vi "InsertBehavior.vi"(7 "exp_type":string, 8 "error in (no error)":errorcluster, 9 "beh_path":path, 10 "beh_start_time":timestamp, 11 "connection reference":T1) -> (0 "error out":errorcluster, 3 "BehaviorPK":T2)   [LabVIEW 2010]
uses:
  <vilib>/addons/database/NI_Database_API.lvlib
  BehPrimary.ctl
  SessionPrimary.ctl
  <vilib>/addons/database/Connection.llb/Conn ObjectReference.ctl
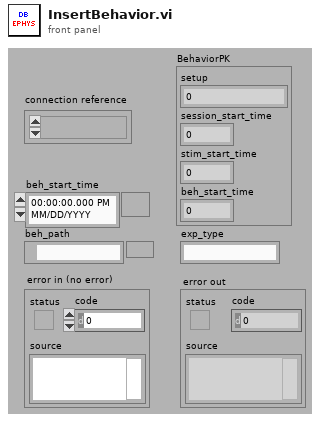
[diagram p1: front panel]
types:
  T1 = typedef "NI_Database_API.lvlib/Conn ObjectReference.ctl" = refnum<k1>
  T2 = typedef "BehPrimary.ctl" = cluster{"setup":u8, "session_start_time":dbl, "stim_start_time":dbl, "beh_start_time":dbl}
  T3 = cluster{"setup":u8, "session_start_time":timestamp, "beh_start_time":timestamp, "beh_path":path, "exp_type":string}
  T4 = typedef "SessionPrimary.ctl" = cluster{"setup":u8, "session_start_time":dbl}
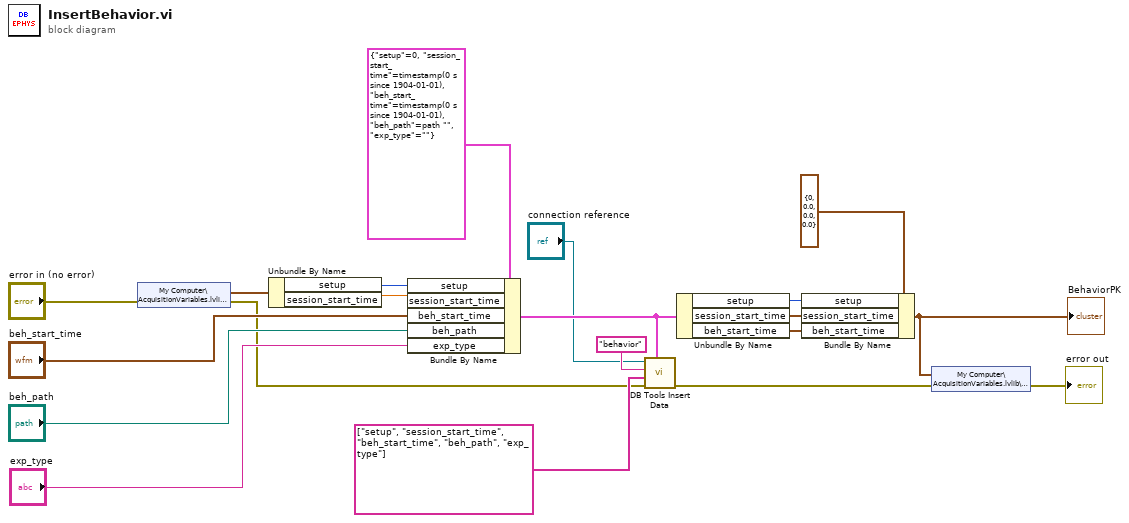
[diagram p0: block diagram]
diagram:
  n1 = shared-variable "My Computer\\AcquisitionVariables.lvlib\\SessionPK"(error in="error in (no error)") -> (w6:T4, error out=w4:errorcluster)
  n2 = Unbundle By Name(w6) -> ("setup"=w17:u8, "session_start_time"=w16:dbl)
  n3 = Bundle By Name(cluster=T3 {"setup"=0, "session_start_time"=timestamp(0 s since 1904-01-01), "beh_start_time"=timestamp(0 s since 1904-01-01), "beh_path"=path "", "exp_type"=""} ("Cluster"), "setup"=w17, "session_start_time"=w16, "beh_start_time"="beh_start_time", "beh_path"="beh_path", "exp_type"="exp_type") -> (w13:T3)
  n4 = call <vilib>:"DB Tools Insert Data.vi"("data"=w13, "error in (no error)"=w4, "columns"=string[] ["setup", "session_start_time", "beh_start_time", "beh_path", "exp_type"], "table"="behavior", "connection reference"="connection reference") -> ("error out"=w2:errorcluster)  [unwired: 5 in, 1 out]
  n5 = Unbundle By Name(w13) -> ("setup"=w12:u8, "session_start_time"=w11:timestamp, "beh_start_time"=w10:timestamp)
  n6 = Bundle By Name(cluster=T2 {"setup"=0, "session_start_time"=0.0, "stim_start_time"=0.0, "beh_start_time"=0.0} ("BehaviorPK"), "setup"=w12, "session_start_time"=w11, "beh_start_time"=w10) -> (w3:T2)
  "BehaviorPK" <- w3
  n7 = shared-variable "My Computer\\AcquisitionVariables.lvlib\\BehaviorPK"(w3, error in=w2) -> (error out=→"error out":errorcluster)
